vi "Initial Path Plot Sub_VI.vi"(10 "Motion Inputs":T4) -> (1 "Accel Array":dbl[](graph), 2 "Velocity Array":dbl[](graph), 3 "Displacement Array":dbl[](graph), 5 "Motion Profile":T1=enum."Triangular", 7 "Motion Outputs":T3)   [LabVIEW 2017]
uses:
  Motion Type Def.ctl
panel:
  out "Motion Planning Outputs":T2
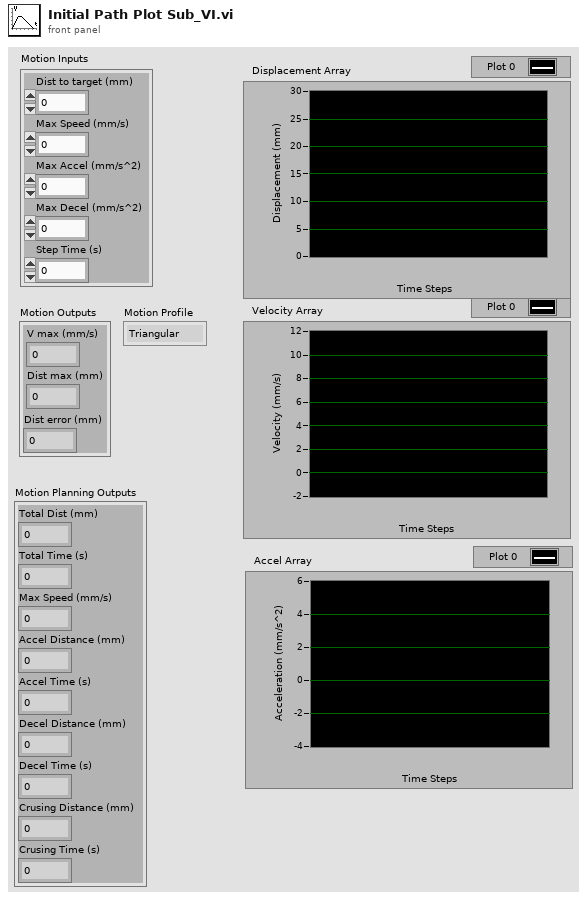
[diagram p1: front panel]
types:
  T1 = typedef "Motion Type Def.ctl" = enum16{"Trapezodial", "Triangular"}
  T2 = cluster{"Crusing Time (s)":dbl, "Decel Time (s)":dbl, "Accel Time (s)":dbl, "Total Time (s)":dbl, "Accel Distance (mm)":dbl, "Decel Distance (mm)":dbl, "Crusing Distance (mm)":dbl, "Total Dist (mm)":dbl, "Max Speed (mm/s)":dbl}
  T3 = cluster{"V max (mm/s)":dbl, "Dist max (mm)":dbl, "Dist error (mm)":dbl}
  T4 = cluster{"Dist to target (mm)":dbl, "Max Speed (mm/s)":dbl, "Max Accel (mm/s^2)":dbl, "Max Decel (mm/s^2)":dbl, "Step Time (s)":dbl}
  T5 = cluster{"Decel Time (s)":dbl, "Accel Time (s)":dbl, "Total Time (s)":dbl, "Accel (mm/s^2)":dbl, "Decel (mm/s^2)":dbl, "Time step (s)":dbl}
  T6 = cluster{" Distance target (mm)":dbl, "Max Accel (mm/s^2)":dbl, "Max Decel (mm/s^2)":dbl, "Velocity Limit (mm/s) ":dbl}
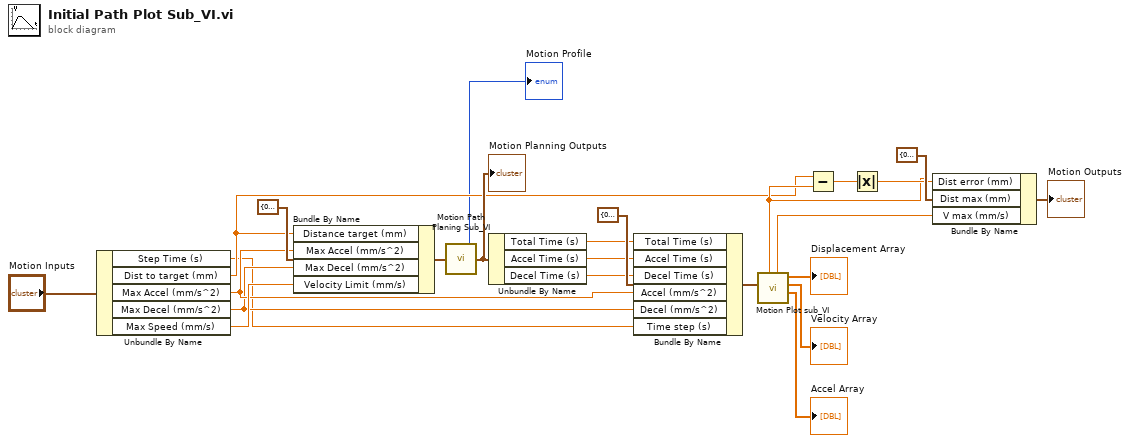
[diagram p0: block diagram]
diagram:
  n1 = Unbundle By Name("Motion Inputs") -> ("Step Time (s)"=w2:dbl, "Dist to target (mm)"=w9:dbl, "Max Accel (mm/s^2)"=w4:dbl, "Max Decel (mm/s^2)"=w3:dbl, "Max Speed (mm/s)"=w20:dbl)
  n2 = Bundle By Name(cluster=T6 {" Distance target (mm)"=0.0, "Max Accel (mm/s^2)"=0.0, "Max Decel (mm/s^2)"=0.0, "Velocity Limit (mm/s) "=0.0} ("Motion Planning Inputs"), "Distance target (mm)"=w9, "Max Accel (mm/s^2)"=w4, "Max Decel (mm/s^2)"=w3, "Velocity Limit (mm/s)"=w20) -> (w18:T6)
  n3 = call "Motion Path Planing Sub_VI.vi"("Motion Planning Inputs"=w18) -> ("Motion Profile"=→"Motion Profile":T1, "Motion Planning Outputs"=w16:T2)  [unwired: 5 in]
  "Motion Planning Outputs" <- w16
  n4 = Unbundle By Name(w16) -> ("Total Time (s)"=w7:dbl, "Accel Time (s)"=w6:dbl, "Decel Time (s)"=w5:dbl)
  n5 = Bundle By Name(cluster=T5 {"Decel Time (s)"=0.0, "Accel Time (s)"=0.0, "Total Time (s)"=0.0, "Accel (mm/s^2)"=0.0, "Decel (mm/s^2)"=0.0, "Time step (s)"=0.01} ("Motion Parameters"), "Total Time (s)"=w7, "Accel Time (s)"=w6, "Decel Time (s)"=w5, "Accel (mm/s^2)"=w4, "Decel (mm/s^2)"=w3, "Time step (s)"=w2) -> (w14:T5)
  n6 = call "Motion Plot sub_VI.vi"("Motion Parameters"=w14) -> ("Acceleration"=→"Accel Array":dbl[], "Velocity"=→"Velocity Array":dbl[], "Displacement"=→"Displacement Array":dbl[], "V max (mm/s)"=w8:dbl, "Dist max (mm)"=w10:dbl)  [unwired: 4 in]
  n7 = Subtract(x=w9, y=w10) -> (x-y=w23:dbl)
  n8 = Absolute Value(x=w23) -> (abs(x)=w19:dbl)
  n9 = Bundle By Name(cluster=T3 {"V max (mm/s)"=0.0, "Dist max (mm)"=0.0, "Dist error (mm)"=0.0} ("Motion Outputs 2"), "Dist error (mm)"=w19, "Dist max (mm)"=w10, "V max (mm/s)"=w8) -> (→"Motion Outputs":T3)
